vi "MAIN_init_queue.vi"(4 "Camera":bool, 5 "error in":errorcluster, 6 "queue MAIN":refnum<queue>, 7 "Start acquisition":bool) -> (1 "error out":errorcluster, 2 "Next task":T1)   [LabVIEW 2015]
uses:
  CONTROLS/Q_main_element.ctl
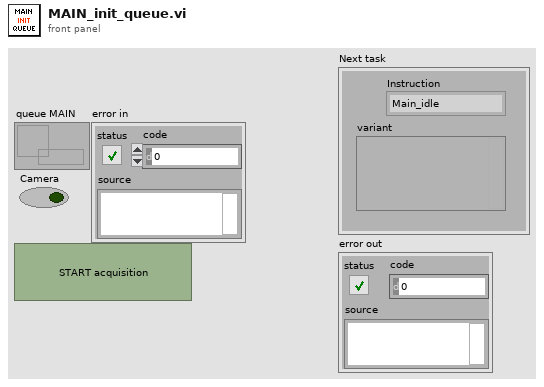
[diagram p1: front panel]
types:
  T1 = typedef "Q_main_element.ctl" = cluster{"variant":variant, "Instruction":enum16{"Main_idle", "Main_initialize", "Main_initialize_TDMS", "Main_initialize_Queue", "Main_error", "Main_DAQ_initialization_results", "Main_ASI_initialization_results", "Main_Piezo_initialization_results", "Main_Valve_initialization_results", "Main_Pump_initialization_results", "Main_CAMERA_initialization_results", "Main_FPGA_initialization_results", "Main_DAQ_error", "Main_ASI_error", "Main_Piezo_error", "Main_CAMERA_error", "Main_Valve_error", "Main_Pump_error", "Main_FPGA_error", "Main_start_acquiring", "Main_not_acquiring", "Main_acquiring", "Main_stop_acquiring", "Main_change_exposure", "Main_change_z_scan_parameters", "Main_define_ROI", "Main_define_mosaic", "Main_read_kinetic_time", "Main_cooler", "Main_read_temperature", "Main_save_XY", "Main_load_XY", "Main_discard_XY", "Main_move_to_XY", "Main_measure_QPD", "Main_autofocus_calibration", "Main_autofocus_initialization", "Main_autofocus_stop", "Main_save_PID", "Main_change_H_valve_position", "Main_two_way_valve", "Main_save_movie", "Main_init_single_scan", "Main_single_scan", "Main_stop_single_scan", "Main_merFISH_illumination_parameters", "Main_merFISH_buffer_probe_list", "Main_merFISH_injections_procedure", "Main_merFISH_save_setpoint", "Main_merFISH_DAPI_parameters", "Main_merFISH_Brightfield_parameters", "Main_merFISH_save_embryo_ROI", "Main_merFISH_init", "Main_merFISH_resume", "Main_merFISH_start_autofocus", "Main_merFISH_open_close_valve_merFISH", "Main_merFISH_open_close_valve_photobleaching", "Main_merFISH_hybridization", "Main_merFISH_move_to_ROI", "Main_merFISH_wait_stabilization", "Main_merFISH_move_to_REF", "Main_merFISH_scan", "Main_merFISH_photobleaching_injection", "Main_merFISH_photobleaching", "Main_merFISH_send_email", "Main_merFISH_close", "Main_STOP"}}
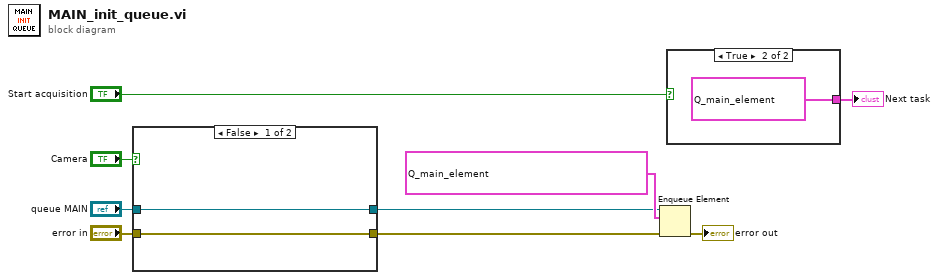
[diagram p0: block diagram]
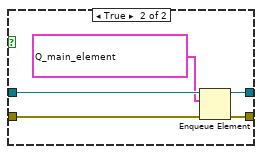
[diagram p2: hidden frame]
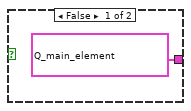
[diagram p3: hidden frame]
diagram:
  n1 = case shown="False" "Camera" {
    tunnel: "error in" -> [w10 w16]
    tunnel: "queue MAIN" -> [w11 w15]
    tunnel: [w10 w13] -> w7
    tunnel: [w11 w12] -> w8
    frame False {
    }
    frame True {
      n2 = Enqueue Element(queue=w15, element=T1 {"variant"=variant, "Instruction"=enum."Main_change_exposure"} ("Q_main_element"), error in (no error)=w16) -> (queue out=w12:refnum<queue>, error out=w13:errorcluster)  [unwired: 1 in, 1 out]
    }
  }
  n3 = Enqueue Element(queue=w8, element=T1 {"variant"=variant, "Instruction"=enum."Main_merFISH_illumination_parameters"} ("Q_main_element"), error in (no error)=w7) -> (error out=→"error out":errorcluster)  [unwired: 1 in, 2 out]
  n4 = case shown="True" "Start acquisition" {
    tunnel: [T1 {"variant"=variant, "Instruction"=enum."Main_not_acquiring"} ("Q_main_element") T1 {"variant"=variant, "Instruction"=enum."Main_acquiring"} ("Q_main_element")] -> w2
    frame False {
    }
    frame True {
    }
  }
  "Next task" <- w2
